vi "Open_Instr.vi"(8 "error in (no error)":errorcluster caption="entrée d'erreur (pas d'erreur)", 11 "Class Multimeter (Default) en entrée":refnum<class "Class Instrument (Default).lvclass">) -> (0 "error out":errorcluster caption="sortie d'erreur", 3 "Class Multimeter (Default) en sortie":refnum<class "Class Instrument (Default).lvclass">)   [LabVIEW 2020, in "Library Instrument & Equipement.lvlib" / "Library Instruments.lvlib" / "Class Instrument (Default).lvclass"]
doc: "Opens and acquires an instrument"
uses:
  Class Instrument (Default).lvclass
  Class Instrument (Default).lvclass/Class Instrument (Default).ctl
  Commun VI/TypeDef/Liste Error.ctl
  Commun VI/Library Commun.lvlib
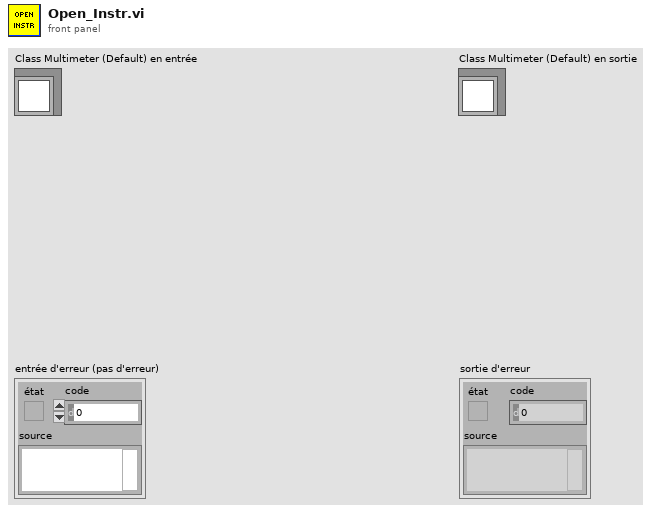
[diagram p1: front panel]
types:
  T1 = typedef "Library Commun.lvlib/Liste Error.ctl" = enum16{"Firebase Driver - Get Document", "Firebase Driver - Get Document With Where", "Firebase Driver - Delete Document", "Firebase Driver - Set Document", "Firebase Driver - Update Document", "Firebase Altyor - Search Document Bench", "Firebase Altyor - Class Not in Firebase", "Spectrum_Analyser - Timeout", "Relay Board - Qty Relay", "DIO - Pb Funtion", "Power_Supply - Peripherical not find", "Mutimeter - Peripherical not find", "Instrument - Function Not Used", "Instrument - Instrument name not specified", "Instrument - Allready Initialised", "Instrument - TimeOut", "Instrument - the instrument must be Initialise before", "Instrument - Frame Not received", "Instrument - Frame Nok", "Test - Initialise the File_for_Save", "Test - Timeout", "Test - Cmd Error", "FGV - Variable ", "BDD FireBase - Define Class", "SN - Class Not Define"}
  T2 = typedef "Semaphore RefNum" = refnum<k1>
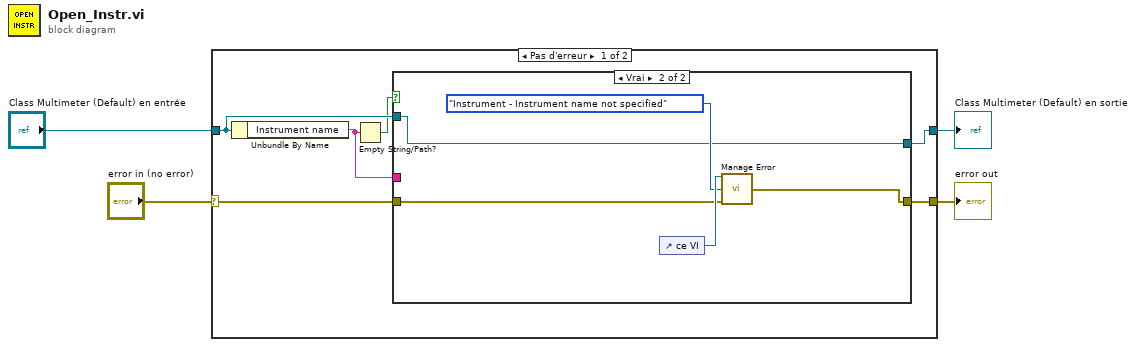
[diagram p0: block diagram]
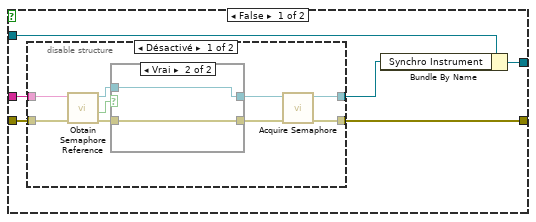
[diagram p2: hidden frame]
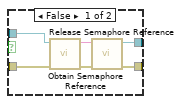
[diagram p3: hidden frame]
diagram:
  n1 = case shown="Pas d'erreur" "error in (no error)" {
    selector: "error in (no error)" -> [w10 w41]
    tunnel: [w8 w41] -> w3
    tunnel: [w9 w40] -> w1
    tunnel: "Class Multimeter (Default) en entrée" -> [w7 w40]
    frame No Error {
      n2 = Unbundle By Name(w7) -> ("Instrument name"=w6:string)
      n3 = Empty String/Path?(string/path=w6) -> (empty?=w5:bool)
      n4 = case shown="Vrai" w5 {
        tunnel: w10 -> [w16 w35]
        tunnel: [w15 w37] -> w9
        tunnel: [w14 w36] -> w8
        tunnel: w7 -> [w12 w37]
        tunnel: w6 -> [w11 _]
        frame False {
          n5 = disable-structure shown="Désactivé" {
            disable-tunnel: w16 -> [w25 w34]
            disable-tunnel: [w21 w34] -> w14
            disable-tunnel: [w19 _] -> w13
            disable-tunnel: w11 -> [w18 _]
            frame Disabled {
              n6 = call <vilib>:"Obtain Semaphore Reference.vi"("error in (no error)"=w25, "name (unnamed)"=w18) -> ("error out"=w17:errorcluster, "created new"=w23:bool, "semaphore"=w24:T2)  [unwired: 3 in]
              n7 = case shown="Vrai" w23 {
                tunnel: w17 -> [w26 w33]
                tunnel: [w27 w33] -> w22
                tunnel: w24 -> [w31 w32]
                tunnel: [w28 w32] -> w20
                frame False {
                  n8 = call <vilib>:"Release Semaphore Reference.vi"("error in (no error)"=w26, "semaphore"=w31) -> ("error out"=w30:errorcluster, "semaphore name"=w29:string)  [unwired: 8 in]
                  n9 = call <vilib>:"Obtain Semaphore Reference.vi"("error in (no error)"=w30, "name (unnamed)"=w29) -> ("error out"=w27:errorcluster, "semaphore"=w28:T2)  [unwired: 3 in, 1 out]
                }
                frame True {
                }
              }
              n10 = call <vilib>:"Acquire Semaphore.vi"("error in (no error)"=w22, "semaphore"=w20) -> ("error out"=w21:errorcluster, "semaphore out"=w19:T2)  [unwired: 3 in, 1 out]
            }
            frame Enabled {
            }
          }
          n11 = Bundle By Name(cluster=w12, "Synchro Instrument"=w13) -> (w15:refnum<class "Class Instrument (Default).lvclass">)
        }
        frame True {
          n12 = control-ref of="ce VI"() -> (w39:refnum<vi>)
          n13 = call "Manage Error.vi"("VI in Error"=w39, "Code Erreur"=Liste_Error."Instrument - Instrument name not specified", "error in (no error)"=w35) -> ("error out"=w36:errorcluster)  [unwired: 12 in]
        }
      }
    }
    frame Error {
    }
  }
  "error out" <- w3
  "Class Multimeter (Default) en sortie" <- w1
